vi "OpenConnection_String.vi"(8 "error in (no error)":errorcluster, 9 "type":string, 10 "topicName":string) -> (0 "error out":errorcluster, 3 "reference":refnum<vi>)   [LabVIEW 2012]
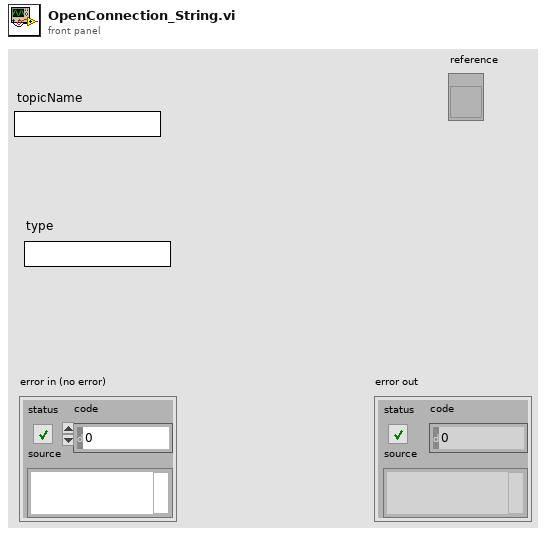
[diagram p1: front panel]
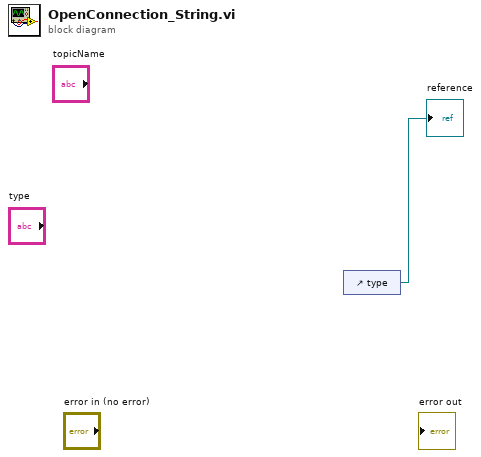
[diagram p0: block diagram]
diagram:
  n1 = control-ref of="type"() -> (→"reference":refnum<vi>)
